vi "TermTypeToString.vi"(11 "Terminal in":refnum<vi>) -> (3 "Name":string)   [LabVIEW 2017]
uses:
  <vilib>/Utility/Data Type/NI_Data Type.lvlib
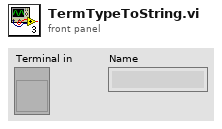
[diagram p1: front panel]
types:
  T1 = typedef "NI_Data Type.lvlib/Data Type.ctl" = enum8{"Invalid Type", "Void", "I8", "I16", "I32", "I64", "U8", "U16", "U32", "U64", "Single Float", "Double Float", "Extended Float", "Single Complex", "Double Complex", "Extended Complex", "Enum U8", "Enum U16", "Enum U32", "Enum U64", "Single Float With Unit", "Double Float With Unit", "Extended Float With Unit", "Single Complex with Unit", "Double Complex with Unit", "Extended Complex with Unit", "Boolean", "String", "Path", "Picture", "Tag", "Array", "Cluster", "Variant", "LV Variant", "Waveform", "Timestamp", "Digital Waveform", "Digital Data", "ExpressData", "Refnum", "External Data", "VI", "Poly VI", "LabVIEW Class Instance", "Fixed Point"}
  T2 = typedef "NI_Data Type.lvlib/Type Definition Info.ctl" = cluster{"Name":string, "Timestamp":u32}
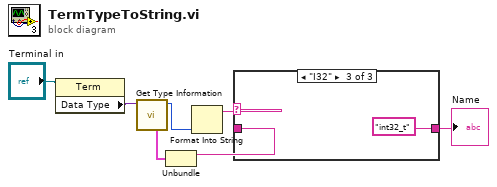
[diagram p0: block diagram]
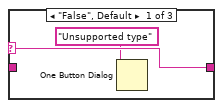
[diagram p2: hidden frame]
diagram:
  n1 = property class="Term"(reference="Terminal in") -> ("Data Type"=w1:variant)  [unwired: 1 in, 2 out]
  n2 = call <vilib>:"Get Type Information.vi"("Variant"=w1) -> ("Type"=w2:T1, "Type Definition Info"=w3:T2)  [unwired: 6 in, 3 out]
  n3 = Unbundle(w3) -> ("Name"=w5:string)  [unwired: 1 out]
  n4 = Format Into String(w2) -> (resulting string=w4:string)  [unwired: 3 in, 1 out]
  n5 = case shown="\"I32\"" w4 {
    selector: w4 -> [w9 _ _]
    tunnel: w5 -> [_ w10 _]
    tunnel: [w9 w10 "int32_t" ("Name")] -> w6
    frame "False", Default {
      n6 = One Button Dialog(message="Unsupported type") -> ()  [unwired: 1 in, 1 out]
    }
    frame "Cluster" {
    }
    frame "I32" {
    }
  }
  "Name" <- w6
